vi "(14) part 2 que.vi"() -> ()   [LabVIEW 2025]
panel:
  out "Numeric 2":dbl
  in  "Numeric":dbl
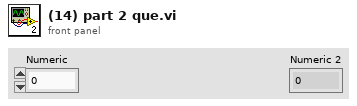
[diagram p1: front panel]
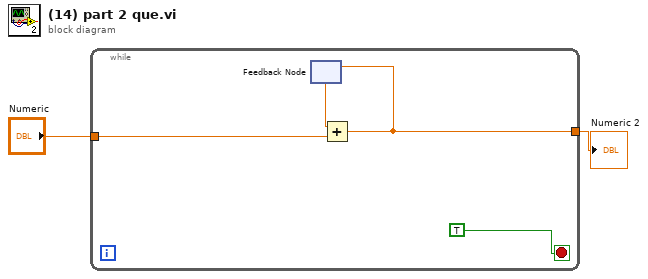
[diagram p0: block diagram]
diagram:
  n1 = while {
    tunnel: "Numeric" -> [w6]
    tunnel: [w5] -> w1
    stop <- TRUE stop-if-true
    n2 = feedback #1() -> (w4:dbl)  [unwired: 1 in]
    n3 = Add(x=w4, y=w6) -> (x+y=w5:dbl)
    n4 = feedback-in #1(w5) -> ()
  }
  "Numeric 2" <- w1
